vi "init.vi"(8 "error in (no error)":errorcluster, 11 "RIOHandler in":refnum<class "RIOHandler.lvclass">) -> (0 "error out":errorcluster, 3 "RIOHandler out":refnum<class "RIOHandler.lvclass">)   [LabVIEW 2013, in "ComponentData.lvlib" / "RIOHandler.lvclass"]
uses:
  <userlib>/Common/Component/common_application/RT/ComponentData/RIOHandler/RIOHandler.lvclass
  <userlib>/Common/Component/common_application/RT/ComponentData/RIOHandler/RIOHandler.lvclass/RIOHandler.ctl
  <userlib>/Common/Component/common_application/RT/ComponentData/ConfigurationHandler/RIOConfig/RIOConfig.lvclass
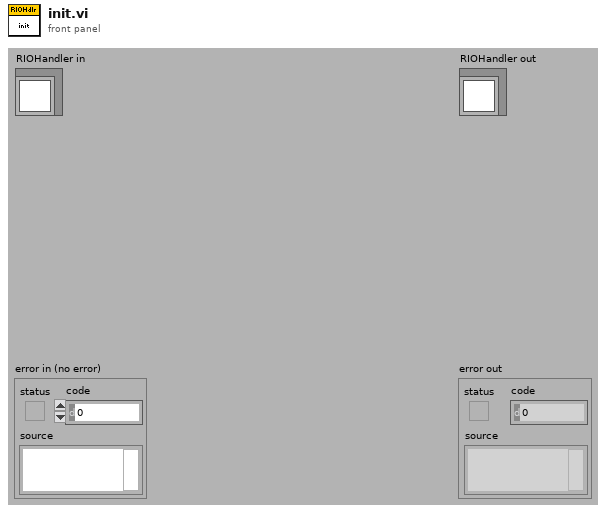
[diagram p1: front panel]
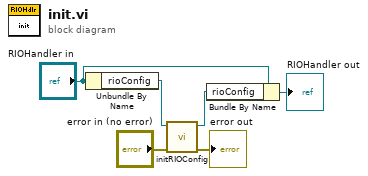
[diagram p0: block diagram]
diagram:
  n1 = Unbundle By Name("RIOHandler in") -> ("rioConfig"=w2:refnum<class "RIOConfig.lvclass">)
  n2 = call <userlib>:"initRIOConfig.vi"("error in (no error)"="error in (no error)", "RIOConfig in"=w2) -> ("error out"=→"error out":errorcluster, "RIOConfig out"=w1:refnum<class "RIOConfig.lvclass">)  [unwired: 8 in]
  n3 = Bundle By Name(cluster="RIOHandler in", "rioConfig"=w1) -> (→"RIOHandler out":refnum<class "RIOHandler.lvclass">)
